vi "set_parameter.vi"(0 "HGF_VariantDataObject":refnum<class "HGF_VariantDataObject.lvclass">, 2 "Parameter":variant, 3 "typeDescriptor":string, 5 "error in (no error)":errorcluster) -> (14 "dup HGF_VariantDataObject":refnum<class "HGF_VariantDataObject.lvclass">, 19 "error out":errorcluster)   [LabVIEW 2014, in "HGF_BaseClasses.lvlib" / "HGF_VariantDataObject.lvclass"]
doc: "Set Parameter."
uses:
  HGF_VariantDataObject.lvclass
  HGF_VariantDataObject.lvclass/HGF_VariantDataObject.ctl
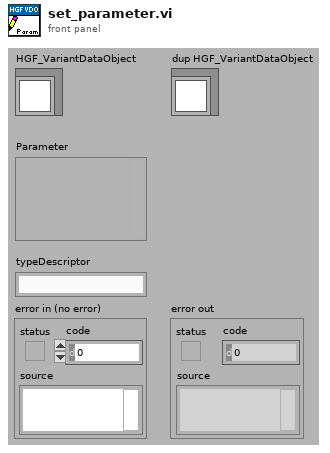
[diagram p1: front panel]
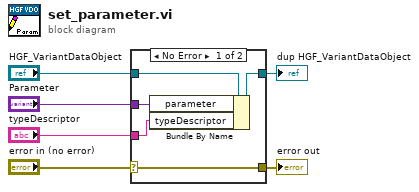
[diagram p0: block diagram]
diagram:
  n1 = case shown="No Error" "error in (no error)" {
    selector: "error in (no error)" -> [w11 w12]
    tunnel: [w11 w12] -> w5
    tunnel: [w9 w13] -> w3
    tunnel: "HGF_VariantDataObject" -> [w10 w13]
    tunnel: "Parameter" -> [w8 _]
    tunnel: "typeDescriptor" -> [w7 _]
    frame No Error {
      n2 = Bundle By Name(cluster=w10, "parameter"=w8, "typeDescriptor"=w7) -> (w9:refnum<class "HGF_VariantDataObject.lvclass">)
    }
    frame Error {
    }
  }
  "error out" <- w5
  "dup HGF_VariantDataObject" <- w3
